vi "Y_H.vi"(8 "error in (no error)":errorcluster, 10 "Change state":bool, 11 "Y_H_in":refnum<class "Y_H.lvclass">) -> (0 "error out":errorcluster, 2 "Change state out":bool, 3 "Y_H_out":refnum<class "Y_H.lvclass">)   [LabVIEW 2019]
uses:
  Sequence/State/State.lvclass
  ctl/Y_H_state.ctl
  Y_H.lvclass
  D:/my_projects/projects/Algorithms/Labview/19/Sequence/State/State.lvclass
panel:
  in  "setpoint":T1(slide) caption="oC" scale=0.0..500.0 scale format="%#_5g"
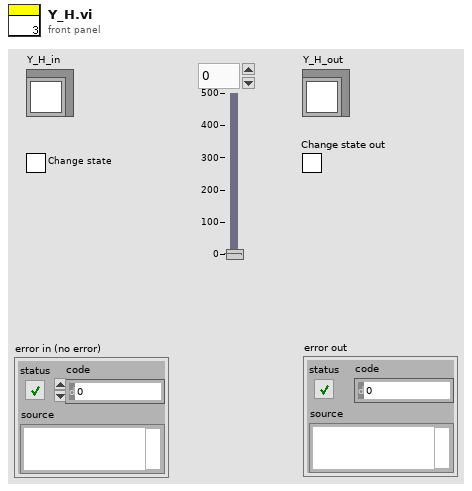
[diagram p1: front panel]
types:
  T1 = cluster{"Numeric":dbl, "Numeric":dbl, "Numeric":dbl}
  T2 = typedef "Y_H.lvclass/Y_H_state.ctl" = enum16{"init", "value change", "value not changed"}
  T3 = enum8{"Enabled", "Disabled", "Disabled and Grayed Out"}
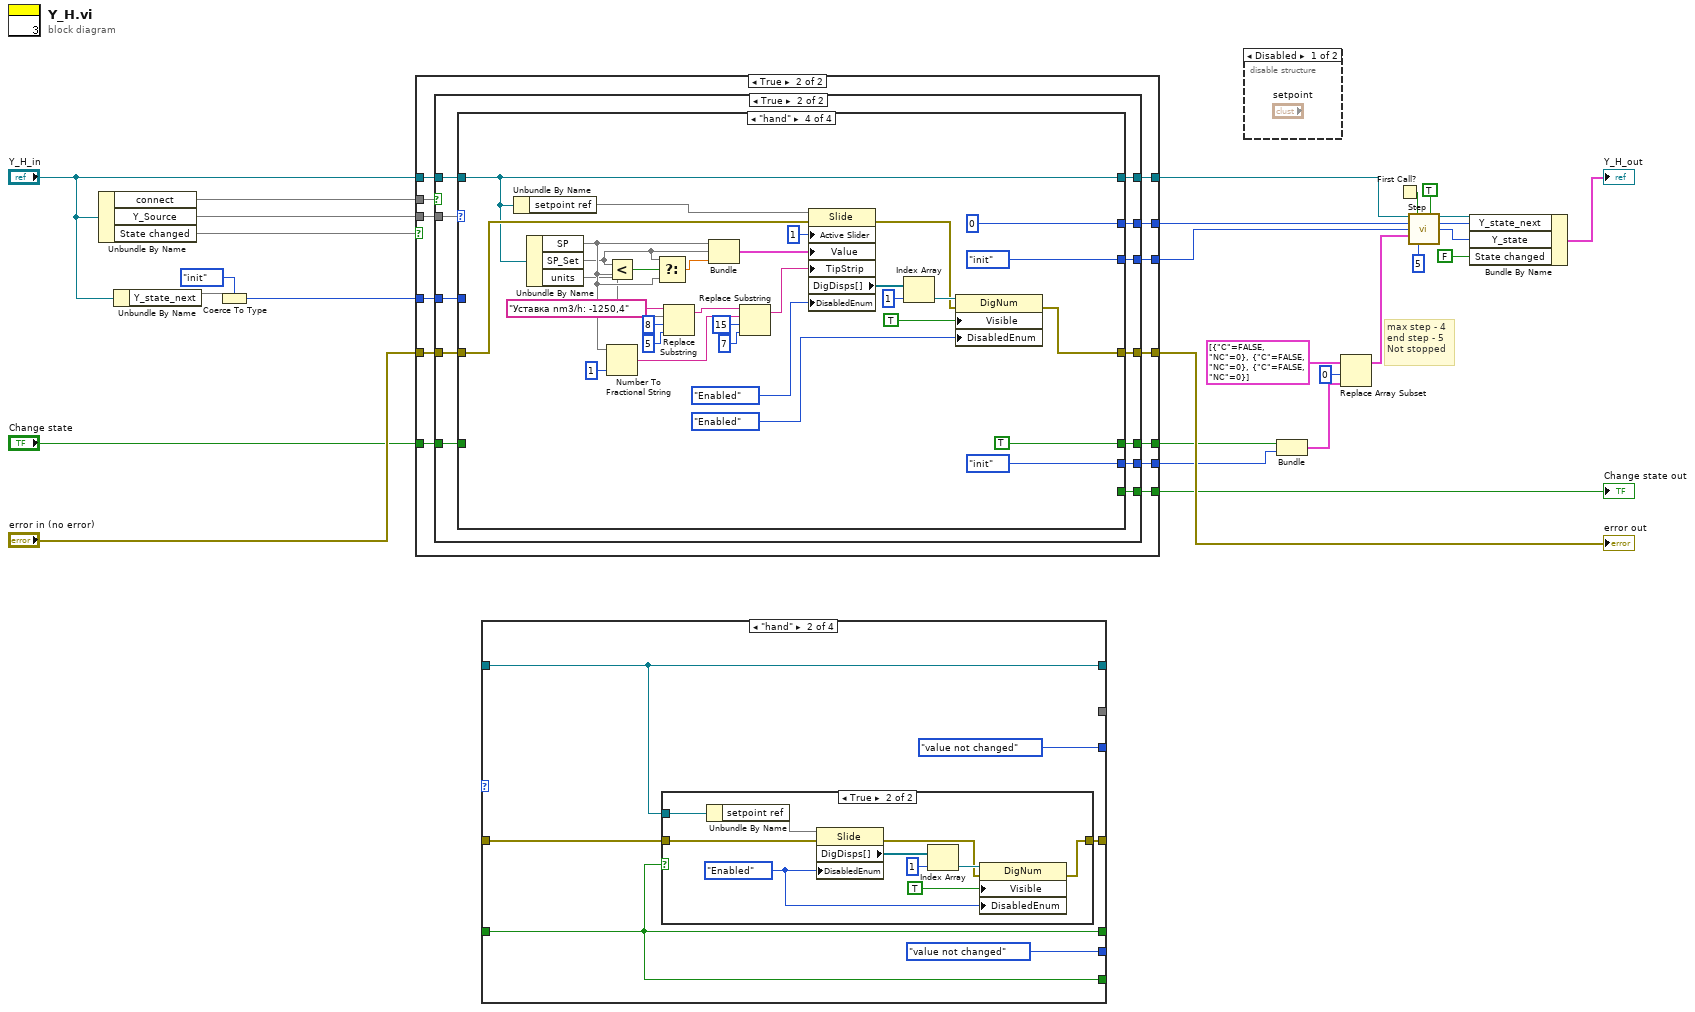
[diagram p0: block diagram]
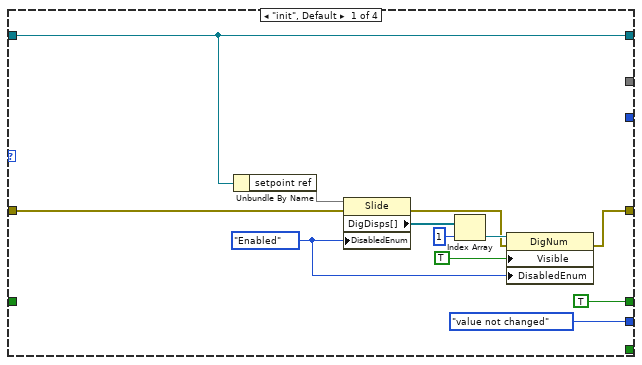
[diagram p2: hidden frame]
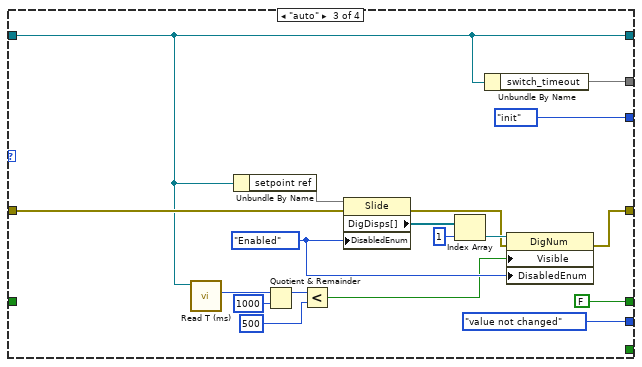
[diagram p4: hidden frame]
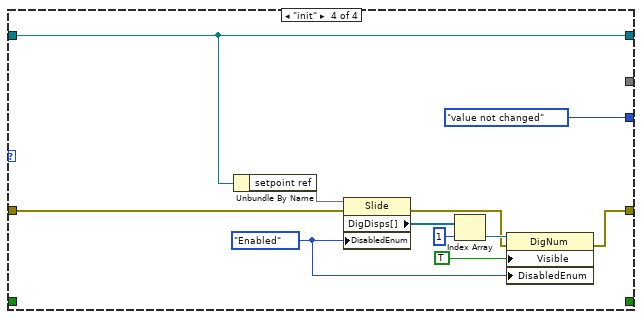
[diagram p5: hidden frame]
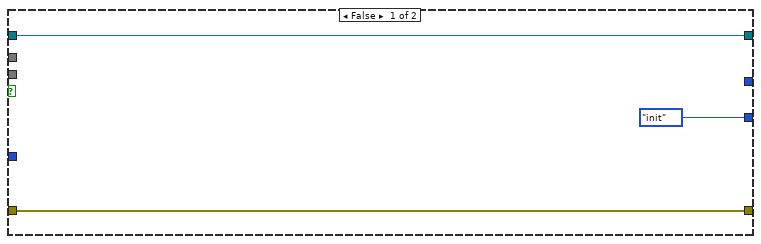
[diagram p6: hidden frame]
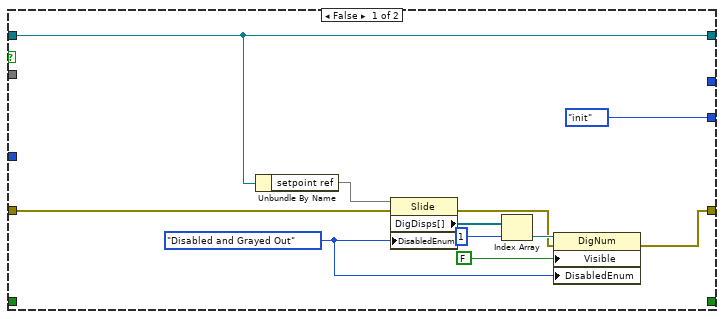
[diagram p7: hidden frame]
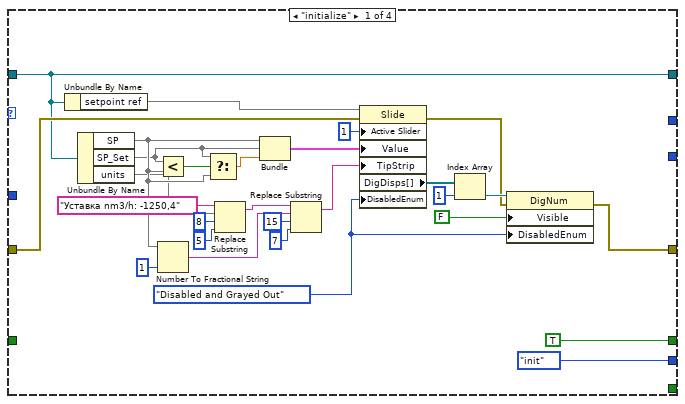
[diagram p8: hidden frame]
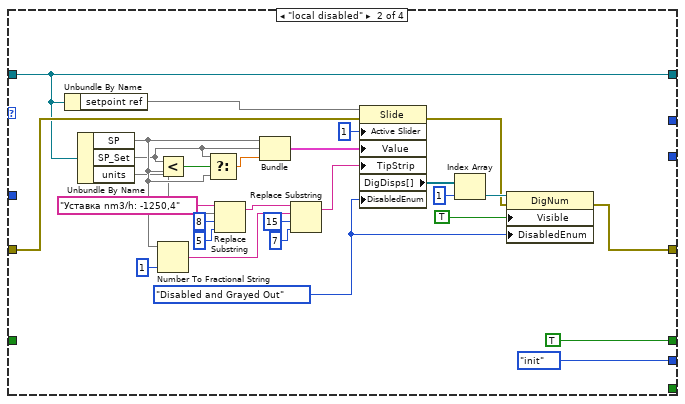
[diagram p9: hidden frame]
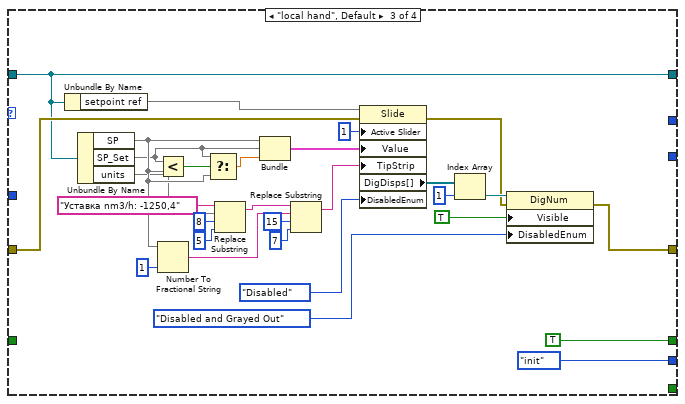
[diagram p10: hidden frame]
diagram:
  # "max step - 4\nend step - 5\nNot stopped"
  n1 = Unbundle By Name("Y_H_in") -> ("connect"=w9, "Y_Source"=w8, "State changed"=w2)
  n2 = Unbundle By Name("Y_H_in") -> ("Y_state_next"=w15)
  n3 = Coerce To Type(0:w15, 1:Y_H_state."init" ("switch_state")) -> (2:w11:T2)
  n4 = case shown="True" w2 {
    tunnel: [Y_H_state."init" ("switch_state") w44] -> w18
    tunnel: "error in (no error)" -> [w29 w43]
    tunnel: [w29 w42] -> w16
    tunnel: [w31 w41] -> w4
    tunnel: [_ w40] -> w1
    tunnel: [_ w39] -> w14
    tunnel: [_ w38] -> w13
    tunnel: w9 -> [_ w37]
    tunnel: "Y_H_in" -> [w31 w36]
    tunnel: w8 -> [_ w35]
    tunnel: w11 -> [_ w34]
    tunnel: "Change state" -> [_ w33]
    tunnel: [_ w32] -> w5
    frame False {
    }
    frame True {
      n5 = case shown="True" w37 {
        tunnel: w35 -> [_ w67]
        tunnel: [w54 w64] -> w41
        tunnel: [Y_H_state."init" ("switch_state") w66] -> w44
        tunnel: w43 -> [w47 w63]
        tunnel: w36 -> [w54 w65]
        tunnel: [w45 w62] -> w42
        tunnel: w34 -> [_ w61]
        tunnel: [_ w60] -> w40
        tunnel: [_ w59] -> w39
        tunnel: [_ w58] -> w38
        tunnel: w33 -> [_ w57]
        tunnel: [_ w56] -> w32
        frame False {
          w50 = T3."Disabled and Grayed Out" ("Disabled")
          n6 = Unbundle By Name(w54) -> ("setpoint ref"=w48)
          n7 = property on="Property Node" class="Slide"(reference=w48, error in=w47, "DisabledEnum"=w50) -> (error out=w46:errorcluster, "DigDisps[]"=w49:refnum<vi>[])  [unwired: 1 out]
          n8 = Index Array(array=w49, index=1) -> (element=w53:refnum<vi>)
          n9 = property class="DigNum"(reference=w53, error in=w46, "Visible"=FALSE ("Z_ASwitch"), "DisabledEnum"=w50) -> (error out=w45:errorcluster)  [unwired: 1 out]
        }
        frame True {
          n10 = case shown="\"hand\"" w67 {
            tunnel: [_ _ _ Y_H_state."init" ("switch_state")] -> w66
            tunnel: w65 -> [w77 w105 w134 w165]
            tunnel: [w77 w105 w134 w165] -> w64
            tunnel: w63 -> [w85 w113 w142 w173]
            tunnel: [w86 w114 w143 w174] -> w62
            tunnel: w61 -> [_ _ _ _]
            tunnel: [_ _ _ u32 0 ("t")] -> w60
            tunnel: [TRUE ("Data") TRUE ("Data") TRUE ("Data") TRUE ("Data")] -> w59
            tunnel: [Y_H_state."init" ("switch_state") Y_H_state."init" ("switch_state") Y_H_state."init" ("switch_state") Y_H_state."init" ("switch_state")] -> w58
            tunnel: w57 -> [_ _ _ _]
            tunnel: [_ _ _ _] -> w56
            frame "initialize" {
              w90 = T3."Disabled and Grayed Out" ("Disabled")
              # "local hand"
              n11 = Unbundle By Name(w77) -> ("setpoint ref"=w88)
              n12 = Unbundle By Name(w77) -> ("SP"=w76, "SP_Set"=w75, "units"=w69)
              n13 = Less?(x=w75, y=w76) -> (x < y?=w83:bool)
              n14 = Number To Fractional String(number=w76, precision (6)=i16 1) -> (F-format string=w70:string)  [unwired: 2 in]
              n15 = Select(t=w75, s=w83, f=w76) -> (s? t:f=w82:dbl)
              n16 = Replace Substring(2:5 ("length (len. of substring)"), 3:8 ("offset (0)"), 4:w69, 5:"Уставка nm3/h: -1250,4") -> (1:w71:string)  [unwired: 1 out]
              n17 = Bundle("SP"=w76, "SP_Set"=w75, w82) -> (w74:cluster{"SP":void, "SP_Set":void, dbl})  [unwired: 1 in]
              n18 = Replace Substring(2:7 ("length (len. of substring)"), 3:15 ("offset (0)"), 4:w70, 5:w71) -> (1:w68:string)  [unwired: 1 out]
              n19 = property on="Property Node" class="Slide"(reference=w88, error in=w85, "Active Slider"=1, "Value"=w74, "TipStrip"=w68, "DisabledEnum"=w90) -> (error out=w87:errorcluster, "DigDisps[]"=w89:refnum<vi>[])  [unwired: 1 out]
              n20 = Index Array(array=w89, index=1) -> (element=w93:refnum<vi>)
              n21 = property class="DigNum"(reference=w93, error in=w87, "Visible"=FALSE ("Z_ASwitch"), "DisabledEnum"=w90) -> (error out=w86:errorcluster)  [unwired: 1 out]
            }
            frame "local disabled" {
              w118 = T3."Disabled and Grayed Out" ("Disabled")
              # "local hand"
              n22 = Unbundle By Name(w105) -> ("setpoint ref"=w116)
              n23 = Unbundle By Name(w105) -> ("SP"=w104, "SP_Set"=w103, "units"=w97)
              n24 = Less?(x=w103, y=w104) -> (x < y?=w111:bool)
              n25 = Number To Fractional String(number=w104, precision (6)=i16 1) -> (F-format string=w98:string)  [unwired: 2 in]
              n26 = Select(t=w103, s=w111, f=w104) -> (s? t:f=w110:dbl)
              n27 = Replace Substring(2:5 ("length (len. of substring)"), 3:8 ("offset (0)"), 4:w97, 5:"Уставка nm3/h: -1250,4") -> (1:w99:string)  [unwired: 1 out]
              n28 = Bundle("SP"=w104, "SP_Set"=w103, w110) -> (w102:cluster{"SP":void, "SP_Set":void, dbl})  [unwired: 1 in]
              n29 = Replace Substring(2:7 ("length (len. of substring)"), 3:15 ("offset (0)"), 4:w98, 5:w99) -> (1:w96:string)  [unwired: 1 out]
              n30 = property on="Property Node" class="Slide"(reference=w116, error in=w113, "Active Slider"=1, "Value"=w102, "TipStrip"=w96, "DisabledEnum"=w118) -> (error out=w115:errorcluster, "DigDisps[]"=w117:refnum<vi>[])  [unwired: 1 out]
              n31 = Index Array(array=w117, index=1) -> (element=w121:refnum<vi>)
              n32 = property class="DigNum"(reference=w121, error in=w115, "Visible"=TRUE ("Z_ASwitch"), "DisabledEnum"=w118) -> (error out=w114:errorcluster)  [unwired: 1 out]
            }
            frame "local hand", Default {
              # "local hand"
              n33 = Unbundle By Name(w134) -> ("setpoint ref"=w145)
              n34 = Unbundle By Name(w134) -> ("SP"=w133, "SP_Set"=w132, "units"=w126)
              n35 = Less?(x=w132, y=w133) -> (x < y?=w140:bool)
              n36 = Number To Fractional String(number=w133, precision (6)=i16 1) -> (F-format string=w127:string)  [unwired: 2 in]
              n37 = Select(t=w132, s=w140, f=w133) -> (s? t:f=w139:dbl)
              n38 = Replace Substring(2:5 ("length (len. of substring)"), 3:8 ("offset (0)"), 4:w126, 5:"Уставка nm3/h: -1250,4") -> (1:w128:string)  [unwired: 1 out]
              n39 = Bundle("SP"=w133, "SP_Set"=w132, w139) -> (w131:cluster{"SP":void, "SP_Set":void, dbl})  [unwired: 1 in]
              n40 = Replace Substring(2:7 ("length (len. of substring)"), 3:15 ("offset (0)"), 4:w127, 5:w128) -> (1:w125:string)  [unwired: 1 out]
              n41 = property on="Property Node" class="Slide"(reference=w145, error in=w142, "Active Slider"=1, "Value"=w131, "TipStrip"=w125, "DisabledEnum"=T3."Disabled" ("Disabled")) -> (error out=w144:errorcluster, "DigDisps[]"=w146:refnum<vi>[])  [unwired: 1 out]
              n42 = Index Array(array=w146, index=1) -> (element=w150:refnum<vi>)
              n43 = property class="DigNum"(reference=w150, error in=w144, "Visible"=TRUE ("Z_ASwitch"), "DisabledEnum"=T3."Disabled and Grayed Out" ("Disabled")) -> (error out=w143:errorcluster)  [unwired: 1 out]
            }
            frame "hand" {
              # "local hand"
              n44 = Unbundle By Name(w165) -> ("setpoint ref"=w176)
              n45 = Unbundle By Name(w165) -> ("SP"=w164, "SP_Set"=w163, "units"=w157)
              n46 = Less?(x=w163, y=w164) -> (x < y?=w171:bool)
              n47 = Number To Fractional String(number=w164, precision (6)=i16 1) -> (F-format string=w158:string)  [unwired: 2 in]
              n48 = Select(t=w163, s=w171, f=w164) -> (s? t:f=w170:dbl)
              n49 = Replace Substring(2:5 ("length (len. of substring)"), 3:8 ("offset (0)"), 4:w157, 5:"Уставка nm3/h: -1250,4") -> (1:w159:string)  [unwired: 1 out]
              n50 = Bundle("SP"=w164, "SP_Set"=w163, w170) -> (w162:cluster{"SP":void, "SP_Set":void, dbl})  [unwired: 1 in]
              n51 = Replace Substring(2:7 ("length (len. of substring)"), 3:15 ("offset (0)"), 4:w158, 5:w159) -> (1:w156:string)  [unwired: 1 out]
              n52 = property on="Property Node" class="Slide"(reference=w176, error in=w173, "Active Slider"=1, "Value"=w162, "TipStrip"=w156, "DisabledEnum"=T3."Enabled" ("Disabled")) -> (error out=w175:errorcluster, "DigDisps[]"=w177:refnum<vi>[])  [unwired: 1 out]
              n53 = Index Array(array=w177, index=1) -> (element=w181:refnum<vi>)
              n54 = property class="DigNum"(reference=w181, error in=w175, "Visible"=TRUE ("Z_ASwitch"), "DisabledEnum"=T3."Enabled" ("Disabled")) -> (error out=w174:errorcluster)  [unwired: 1 out]
            }
          }
        }
      }
    }
  }
  "error out" <- w16
  "Change state out" <- w5
  n55 = case shown="\"hand\"" {
    selector: _ -> [_ _ _ _]
    tunnel: [w184 w198 w213 w232] -> _
    tunnel: _ -> [w184 w198 w213 w232]
    tunnel: [_ Y_H_state."value not changed" ("switch_state") Y_H_state."init" ("switch_state") Y_H_state."value not changed" ("switch_state")] -> _
    tunnel: _ -> [w186 w199 w216 w233]
    tunnel: [w185 w197 w215 w231] -> _
    tunnel: [_ _ w230 _] -> _
    tunnel: [TRUE ("Data") w196 FALSE ("Data") _] -> _
    tunnel: [Y_H_state."value not changed" ("switch_state") Y_H_state."value not changed" ("switch_state") Y_H_state."value not changed" ("switch_state") _] -> _
    tunnel: _ -> [_ w196 _ _]
    tunnel: [_ w196 _ _] -> _
    frame "init", Default {
      w190 = T3."Enabled" ("Disabled")
      n56 = Unbundle By Name(w184) -> ("setpoint ref"=w188)
      n57 = property on="Property Node" class="Slide"(reference=w188, error in=w186, "DisabledEnum"=w190) -> (error out=w187:errorcluster, "DigDisps[]"=w189:refnum<vi>[])  [unwired: 1 out]
      n58 = Index Array(array=w189, index=1) -> (element=w193:refnum<vi>)
      n59 = property class="DigNum"(reference=w193, error in=w187, "Visible"=TRUE ("Z_ASwitch"), "DisabledEnum"=w190) -> (error out=w185:errorcluster)  [unwired: 1 out]
    }
    frame "hand" {
      n60 = case shown="True" w196 {
        tunnel: w199 -> [w202 w205]
        tunnel: w198 -> [_ w203]
        tunnel: [w202 w204] -> w197
        frame False {
        }
        frame True {
          w209 = T3."Enabled" ("Disabled")
          n61 = Unbundle By Name(w203) -> ("setpoint ref"=w207)
          n62 = property on="Property Node" class="Slide"(reference=w207, error in=w205, "DisabledEnum"=w209) -> (error out=w206:errorcluster, "DigDisps[]"=w208:refnum<vi>[])  [unwired: 1 out]
          n63 = Index Array(array=w208, index=1) -> (element=w212:refnum<vi>)
          n64 = property class="DigNum"(reference=w212, error in=w206, "Visible"=TRUE ("Z_ASwitch"), "DisabledEnum"=w209) -> (error out=w204:errorcluster)  [unwired: 1 out]
        }
      }
    }
    frame "auto" {
      w218 = T3."Enabled" ("Disabled")
      n65 = call "Read T (ms).vi"("State in"=w213) -> ("T (ms)"=w225:u32)  [unwired: 9 in, 1 out]
      n66 = Unbundle By Name(w213) -> ("setpoint ref"=w220)
      n67 = Quotient & Remainder(x=w225, y=u32 1000) -> (x-y*floor(x/y)=w228:u32)  [unwired: 1 out]
      n68 = Less?(x=w228, y=u32 500) -> (x < y?=w214:bool)
      n69 = property on="Property Node" class="Slide"(reference=w220, error in=w216, "DisabledEnum"=w218) -> (error out=w219:errorcluster, "DigDisps[]"=w221:refnum<vi>[])  [unwired: 1 out]
      n70 = Index Array(array=w221, index=1) -> (element=w222:refnum<vi>)
      n71 = Unbundle By Name(w213) -> ("switch_timeout"=w230)
      n72 = property class="DigNum"(reference=w222, error in=w219, "Visible"=w214, "DisabledEnum"=w218) -> (error out=w215:errorcluster)  [unwired: 1 out]
    }
    frame "init" {
      w237 = T3."Enabled" ("Disabled")
      n73 = Unbundle By Name(w232) -> ("setpoint ref"=w235)
      n74 = property on="Property Node" class="Slide"(reference=w235, error in=w233, "DisabledEnum"=w237) -> (error out=w234:errorcluster, "DigDisps[]"=w236:refnum<vi>[])  [unwired: 1 out]
      n75 = Index Array(array=w236, index=1) -> (element=w240:refnum<vi>)
      n76 = property class="DigNum"(reference=w240, error in=w234, "Visible"=TRUE ("Z_ASwitch"), "DisabledEnum"=w237) -> (error out=w231:errorcluster)  [unwired: 1 out]
    }
  }
  n77 = disable-structure shown="Disabled" {
    frame Disabled {
    }
    frame Enabled {
    }
  }
  n78 = Bundle("Data"=w14, "switch_state"=w13) -> (w20:cluster{"Data":bool, "switch_state":T2})  [unwired: 1 in]
  n79 = Replace Array Subset(array=cluster{"C":bool, "NC":u32}[] [{"C"=FALSE, "NC"=0}, {"C"=FALSE, "NC"=0}, {"C"=FALSE, "NC"=0}] ("appended array"), new element=w20, index=0) -> (w19:cluster{"C":bool, "NC":u32}[])
  n80 = First Call?() -> (First Call?: T/F=w28:bool)
  n81 = call "Step.vi"("State in"=w4, "Reset"=w28, "Start in"=TRUE ("Start"), "t"=w1, "Nt"=w18, "C_table"=w19, "N end step"=u32 5) -> ("State out"=w3:refnum<class "Y_H.lvclass">, "N next"=w26:u32, "N curr"=w27:u32)  [unwired: 5 in, 1 out]
  n82 = Bundle By Name(cluster=w3, "Y_state_next"=w26, "Y_state"=w27, "State changed"=FALSE ("Data changed")) -> (→"Y_H_out":cluster{})
